vi "Init Times & Stations Cluster.vi"(8 "error in (no error)":errorcluster) -> (0 "error out":errorcluster, 3 "Times and Stations":T1={"Wash Times"=[5.0, 5.0, 5.0, 5.0, 5.0, 5.0, 5.0, 5.0], "Stations"=[enum."Station 1", enum."Station 1", enum."Station 2", enum."Station 2", enum."Station 2", enum."Station 2", enum."Station 3", enum."Station 3"]})   [LabVIEW 2010]
doc: "This VI just inits the Times and Stations Cluster."
uses:
  Controls/Times and Stations Cluster_TDef.ctl
  Controls/Stations ENUM_TDef.ctl
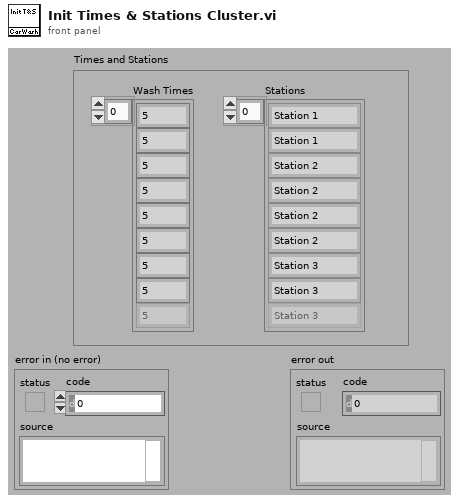
[diagram p1: front panel]
types:
  T1 = typedef "Times and Stations Cluster_TDef.ctl" = cluster{"Wash Times":dbl[], "Stations":T2[]}
  T2 = typedef "Stations ENUM_TDef.ctl" = enum16{"Station 1", "Station 2", "Station 3"}
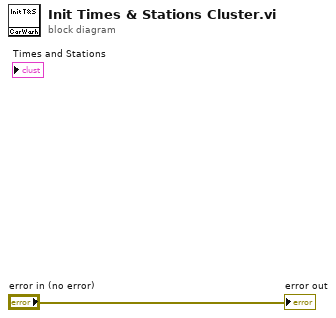
[diagram p0: block diagram]
diagram:
  "error out" <- "error in (no error)"
